vi "Get Root Actors.vi"(8 "error in (no error)":errorcluster, 11 "Monitor Data in":refnum<class "Monitor Data.lvclass">) -> (0 "error out":errorcluster, 2 "Root Actors":refnum<class "Message Enqueuer.lvclass">[](array[class]), 3 "Monitor Data out":refnum<class "Monitor Data.lvclass">)   [LabVIEW 2023, in "Monitored Actor.lvlib" / "Monitor Data.lvclass"]
doc: "Returns the root level actors\n\nCopyright: MGI 2016\nAuthor: Derek Trepanier"
uses:
  Monitor Data.lvclass
  builds/Engine/Actor Framework.lvlibp/1abvi3w/vi.lib/ActorFramework/Message Enqueuer/Message Enqueuer.lvclass
  Monitor Data.lvclass/Monitor Data.ctl
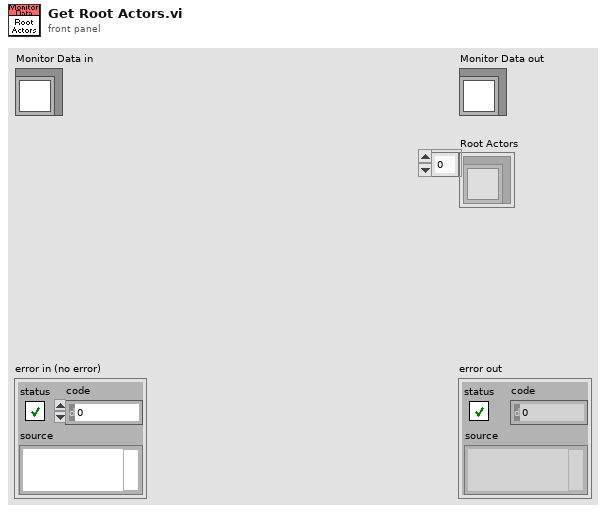
[diagram p1: front panel]
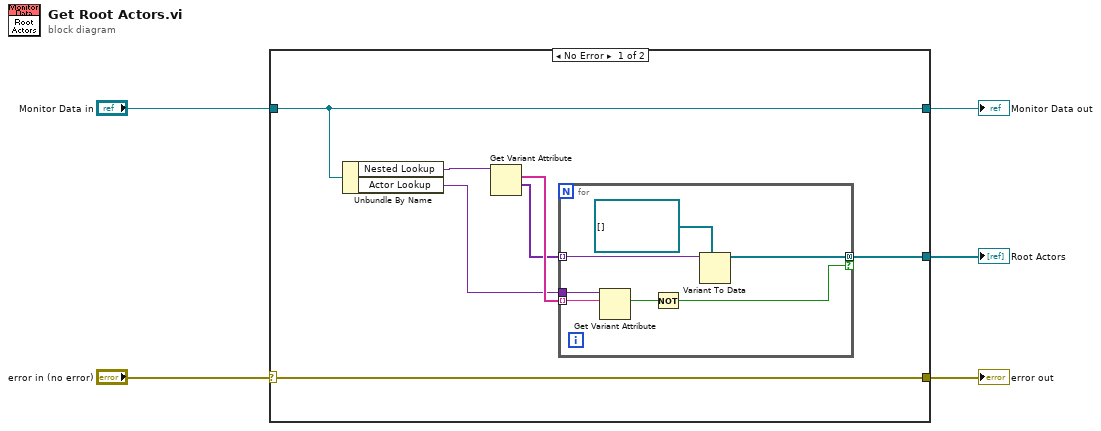
[diagram p0: block diagram]
diagram:
  n1 = case shown="No Error" "error in (no error)" {
    selector: "error in (no error)" -> [w12 w21]
    tunnel: [w12 w21] -> w4
    tunnel: [w11 w20] -> w2
    tunnel: "Monitor Data in" -> [w11 w20]
    tunnel: [w10 _] -> w1
    frame No Error {
      n2 = Unbundle By Name(w11) -> ("Nested Lookup"=w7:variant, "Actor Lookup"=w6:variant)
      n3 = Get Variant Attribute(Variant=w7) -> (names=w9:string[], values=w8:variant[])  [unwired: 3 in, 2 out]
      n4 = for {
        tunnel: w9 -> [w18] mode=indexing
        tunnel: [w14] -> w10 mode=concatenating if=w13
        tunnel: w8 -> [w16] mode=indexing
        tunnel: w6 -> [w19]
        n5 = Get Variant Attribute(Variant=w19, name=w18) -> (found=w17:bool)  [unwired: 2 in, 3 out]
        n6 = Not(x=w17) -> (.not. x?=w13:bool)
        n7 = Variant To Data(type=refnum<class "Message Enqueuer.lvclass">[] [], Variant=w16) -> (data=w14:refnum<class "Message Enqueuer.lvclass">[])  [unwired: 1 in, 1 out]
      }
    }
    frame Error {
    }
  }
  "error out" <- w4
  "Monitor Data out" <- w2
  "Root Actors" <- w1
